vi "Go.vi"(9 "Timing Data":T1(array[cluster]), 10 "Control In":T2={"I-O.lvclass"=refnum, "Gantry"=refnum, "Dispenser"="COM1"}, 11 "C4 Dispense in":refnum<class "Iterative Dispense.lvclass">) -> (2 "Control Out":T2={"I-O.lvclass"=refnum, "Gantry"=refnum, "Dispenser"="COM1"}, 3 "C4 Dispense Out":refnum<class "Iterative Dispense.lvclass">)   [LabVIEW 2018, in "Iterative Dispense.lvclass"]
uses:
  Iterative Dispense.lvclass
  C:/Users/HEP/Documents/GitHub/New folder/C/Users/HEP/Documents/GitHub/UCSB-Gantry-HEP-2018/Classes/Routine/Dispense/Dispense.lvclass
  Controller/Controllers.ctl
  Controller/I-O/I-O.lvclass
  C:/Program Files (x86)/Aerotech/A3200/LabVIEW/2010/Bin/Aerotech.A3200.dll
  Program Files (x86)/Aerotech/A3200/LabVIEW/2010/Bin/Aerotech.A3200.dll
  Iterative Dispense.lvclass/Iterative Dispense.ctl
  Controller/Motion/A3200/A3200.lvclass
  Controller/Dispenser/Dispenser.lvclass
  Controller/Motion/Motion.lvclass
  Controller/Controller.lvclass
panel:
  out "error out":errorcluster
  in  "error in (no error)":errorcluster
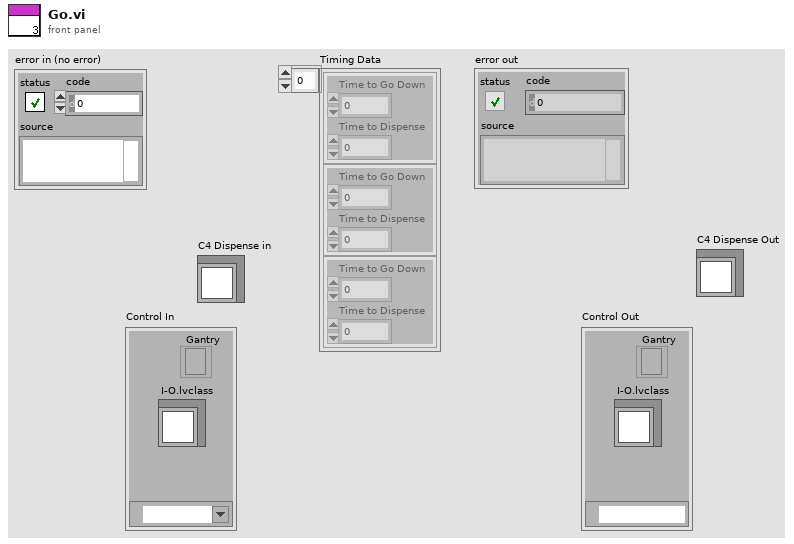
[diagram p1: front panel]
types:
  T1 = cluster{"Time to Go Down":i32, "Time to Dispense":i32}[]
  T2 = typedef "Controller.lvclass/Controllers.ctl" = cluster{"I-O.lvclass":refnum<class "I-O.lvclass">, "Gantry":refnum<k24>, "Dispenser":refnum<visa-resource-name>}
  T3 = typedef "Iterative Dispense.lvclass/Glue Step Enum.ctl" = enum16{"Baseplate to Kapton", "Kapton to Sensor"}
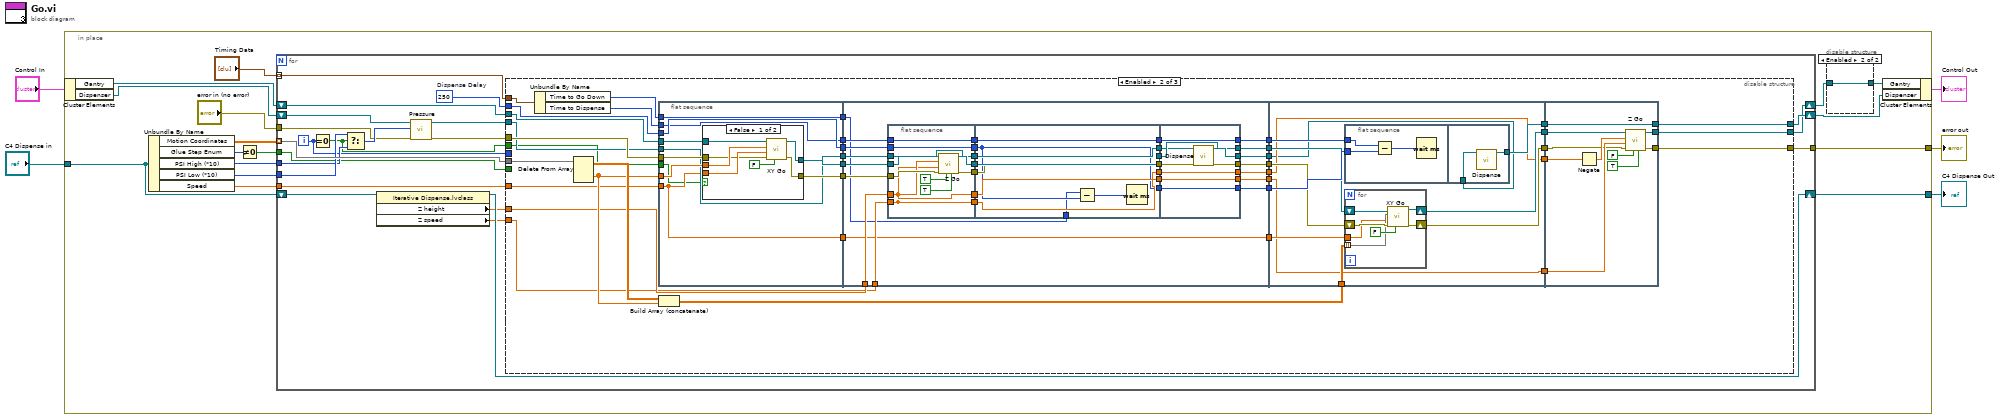
[diagram p0: block diagram]
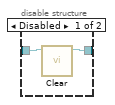
[diagram p2: hidden frame]
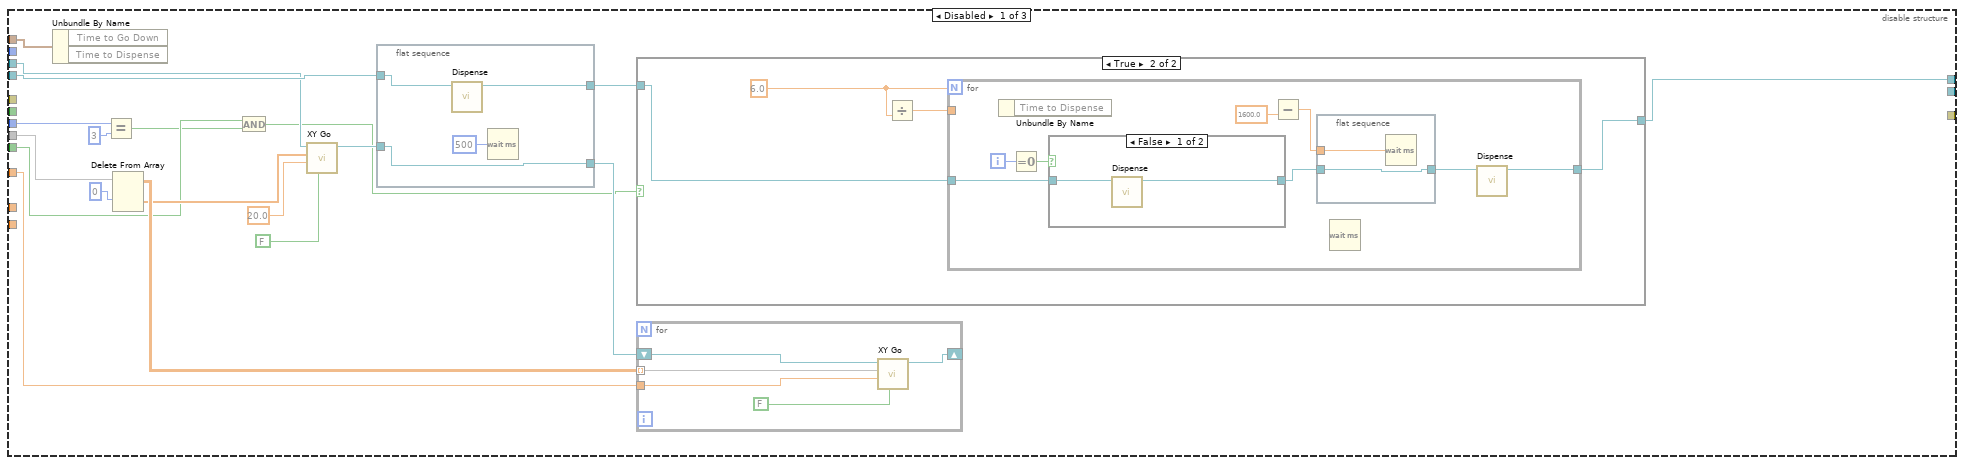
[diagram p3: hidden frame]
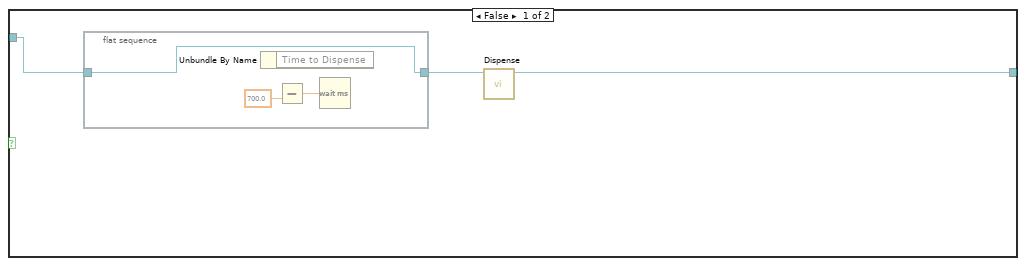
[diagram p4: hidden frame]
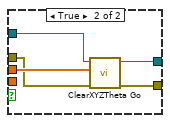
[diagram p6: hidden frame]
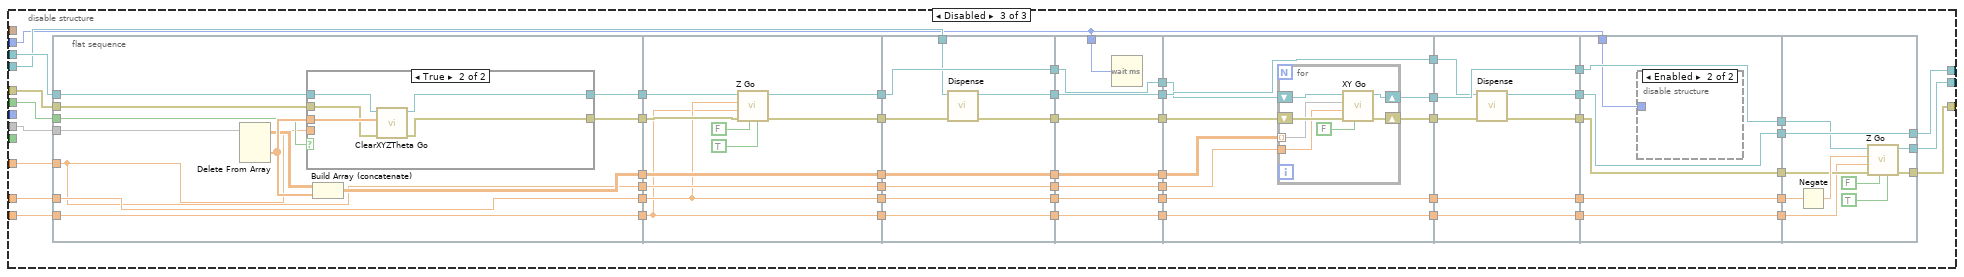
[diagram p7: hidden frame]
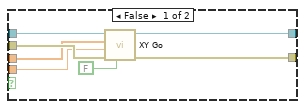
[diagram p8: hidden frame]
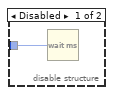
[diagram p9: hidden frame]
diagram:
  n1 = in-place {
    in-place-border: "C4 Dispense in" -> [w9]
    in-place-border: [w10] -> w2
    in-place-border: [w7] -> w1
    n2 = in-place-cluster #1("Control In") -> ("Gantry"=w15:refnum<k24>, "Dispenser"=w13:refnum<visa-resource-name>)
    n3 = Unbundle By Name(w9) -> ("Motion Coordinates"=w17:dbl[][][], "Glue Step Enum"=w16:T3, "PSI High (*10)"=w20:i32, "PSI Low (*10)"=w19:i32, "Speed"=w18:dbl)
    n4 = Not Equal To 0?(x=w16) -> (x != 0?=w21:bool)
    n5 = for {
      tunnel: w17 -> [w45] mode=indexing
      tunnel: w21 -> [w26]
      tunnel: w18 -> [w44]
      tunnel: w19 -> [w43]
      tunnel: w20 -> [w42]
      shift-right: [w28] -> w12
      shift-left: w15 -> [w40]
      shift-right: [w46] -> w14
      shift-left: w13 -> [w39]
      tunnel: "error in (no error)" -> [w36]
      shift-right: [w34] -> w10
      shift-left: w9 -> [w35]
      tunnel: [w30] -> w7
      tunnel: "Timing Data" -> [w27] mode=indexing
      i -> [w25]
      w31 = 250  # Dispense Delay
      # "Executes C4 Symmetric Motion"
      n6 = Equal To 0?(x=w25) -> (x = 0?=w29:bool)
      n7 = Select(t=w43, s=w29, f=w42) -> (s? t:f=w41:i32)
      n8 = property class="Iterative Dispense.lvclass"(reference=w35) -> (reference out=w34:refnum<class "Iterative Dispense.lvclass">, "Z height"=w33:dbl, "Z speed"=w32:dbl)  [unwired: 1 in, 1 out]
      n9 = call "Pressure.vi"("error in (no error)"=w36, "Pressure"=w41, "VISA resource name"=w39) -> ("error out"=w37:errorcluster, "VISA resource name out"=w38:refnum<visa-resource-name>)  [unwired: 7 in]
      n10 = disable-structure shown="Enabled" {
        disable-tunnel: [w65 w109 w285] -> w46
        disable-tunnel: w45 -> [w64 w121 w287]
        disable-tunnel: w44 -> [w59 w118 w304]
        disable-tunnel: w38 -> [w58 w116 w286]
        disable-tunnel: w40 -> [w57 w123 w289]
        disable-tunnel: w37 -> [_ w117 w288]
        disable-tunnel: w33 -> [_ w114 w291]
        disable-tunnel: w32 -> [_ w113 w292]
        disable-tunnel: w31 -> [_ w105 w255]
        disable-tunnel: [_ w108 w284] -> w30
        disable-tunnel: w29 -> [_ w98 w290]
        disable-tunnel: [_ w122 w252] -> w28
        disable-tunnel: w27 -> [w52 w107 _]
        disable-tunnel: w26 -> [w51 _ _]
        disable-tunnel: w25 -> [w50 _ _]
        frame Disabled {
          n11 = Unbundle By Name(w52) -> ()  [unwired: 2 out]
          n12 = Equal?(x=w50, y=3) -> (x = y?=w48:bool)
          n13 = Delete From Array(array=w64, index (row)=0) -> (deleted portion=w55:dbl[], array with subset deleted=w62:dbl[][])  [unwired: 2 in]
          n14 = And(x=w51, y=w48) -> (x .and. y?=w47:bool)
          n15 = call "XY Go.vi"("return immediately"=FALSE, "Speed"=20.0 ("speed"), "XY In"=w55, "Gantry In"=w57) -> ("Gantry Out"=w56:refnum<k24>)  [unwired: 5 in, 2 out]
          n16 = flat-sequence {
            tunnel: w58 -> [w89]
            tunnel: w56 -> [w91]
            tunnel: [w91] -> w61
            tunnel: [w90] -> w60
            frame #0 {
              n17 = call "Dispense.vi"("Dispenser In"=w89) -> ("Dispenser Out"=w90:refnum<visa-resource-name>)  [unwired: 9 in, 1 out]
              n18 = Wait (ms)(milliseconds to wait=u32 500) -> ()  [unwired: 1 out]
            }
          }
          n19 = case shown="True" w47 {
            tunnel: w60 -> [w68 w74]
            tunnel: [w67 w73] -> w65
            frame False {
              n20 = flat-sequence {
                tunnel: w68 -> [w69]
                tunnel: [w69] -> w66
                frame #0 {
                  n21 = Unbundle By Name() -> ()  [unwired: 1 in, 1 out]
                  n22 = Subtract(y=700.0) -> (x-y=w71:dbl)  [unwired: 1 in]
                  n23 = Wait (ms)(milliseconds to wait=w71) -> ()  [unwired: 1 out]
                }
              }
              n24 = call "Dispense.vi"("Dispenser In"=w66) -> ("Dispenser Out"=w67:refnum<visa-resource-name>)  [unwired: 9 in, 1 out]
            }
            frame True {
              w72 = 6.0 ("y")
              # "Leaves Space for Silver Epoxy"
              n25 = Divide(y=w72) -> (x/y=w75:dbl)  [unwired: 1 in]
              n26 = for {
                N: w72 -> [_]
                tunnel: w75 -> [_]
                tunnel: w74 -> [w81]
                tunnel: [w77] -> w73
                i -> [w79]
                n27 = Unbundle By Name() -> ()  [unwired: 1 in, 1 out]
                n28 = Equal To 0?(x=w79) -> (x = 0?=w78:bool)
                n29 = case shown="False" w78 {
                  tunnel: w81 -> [w84 w86]
                  tunnel: [w85 w86] -> w80
                  frame False {
                    n30 = call "Dispense.vi"("Dispenser In"=w84) -> ("Dispenser Out"=w85:refnum<visa-resource-name>)  [unwired: 9 in, 1 out]
                  }
                  frame True {
                  }
                }
                n31 = Subtract(y=1600.0) -> (x-y=w82:dbl)  [unwired: 1 in]
                n32 = flat-sequence {
                  tunnel: w82 -> [w88]
                  tunnel: w80 -> [w87]
                  tunnel: [w87] -> w76
                  frame #0 {
                    n33 = Wait (ms)(milliseconds to wait=w88) -> ()  [unwired: 1 out]
                  }
                }
                n34 = Wait (ms)() -> ()  [unwired: 1 in, 1 out]
                n35 = call "Dispense.vi"("Dispenser In"=w76) -> ("Dispenser Out"=w77:refnum<visa-resource-name>)  [unwired: 9 in, 1 out]
              }
            }
          }
          n36 = for {
            tunnel: w59 -> [w94]
            tunnel: w62 -> [w95] mode=indexing
            shift-right: [w96] -> _
            shift-left: w61 -> [w97]
            n37 = call "XY Go.vi"("return immediately"=FALSE, "Speed"=w94, "XY In"=w95, "Gantry In"=w97) -> ("Gantry Out"=w96:refnum<k24>)  [unwired: 5 in, 2 out]
          }
        }
        frame Enabled {
          n38 = Unbundle By Name(w107) -> ("Time to Go Down"=w102:i32, "Time to Dispense"=w100:i32)
          n39 = Delete From Array(array=w121) -> (deleted portion=w119:dbl[], array with subset deleted=w120:dbl[][])  [unwired: 3 in]
          n40 = flat-sequence {
            tunnel: w123 -> [w146]
            tunnel: [w145] -> w135
            tunnel: [w142] -> w134
            tunnel: w119 -> [w144]
            tunnel: w118 -> [w140]
            tunnel: w117 -> [w143]
            tunnel: w116 -> [w141]
            tunnel: [w141] -> w115
            tunnel: [w140] -> w111
            tunnel: [w139] -> w106
            tunnel: w105 -> [w139]
            tunnel: [w138] -> w103
            tunnel: w102 -> [w138]
            tunnel: [w137] -> w101
            tunnel: w100 -> [w137]
            tunnel: w98 -> [w136]
            tunnel: w135 -> [w187]
            tunnel: [w188] -> w133
            tunnel: [w186] -> w132
            tunnel: w134 -> [w185]
            tunnel: [w183] -> w131
            tunnel: [w182] -> w130
            tunnel: [w181] -> w129
            tunnel: w115 -> [w184]
            tunnel: w114 -> [w180]
            tunnel: w113 -> [w179]
            tunnel: w111 -> [w178]
            tunnel: [w178] -> w110
            tunnel: w106 -> [w177]
            tunnel: [w176] -> w104
            tunnel: w103 -> [w159]
            tunnel: w101 -> [w175]
            tunnel: [w174] -> w99
            tunnel: w133 -> [w218]
            tunnel: [w229] -> w128
            tunnel: w132 -> [w226]
            tunnel: [w222] -> w127
            tunnel: [w220] -> w126
            tunnel: w131 -> [w220]
            tunnel: [w219] -> w125
            tunnel: w130 -> [w219]
            tunnel: w129 -> [w225]
            tunnel: [w221] -> w124
            tunnel: w112 -> [w224]
            tunnel: w110 -> [w223]
            tunnel: w104 -> [w228]
            tunnel: w99 -> [w227]
            tunnel: [w251] -> w122
            tunnel: w128 -> [w250]
            tunnel: [w250] -> w109
            tunnel: w127 -> [w249]
            tunnel: [w248] -> w108
            tunnel: w126 -> [w247]
            tunnel: w125 -> [w245]
            tunnel: w124 -> [w242]
            frame #0 {
              n41 = case shown="False" w136 {
                tunnel: w146 -> [w153 w158]
                tunnel: [w152 w157] -> w145
                tunnel: [w151 w156] -> w142
                tunnel: w144 -> [w149 w155]
                tunnel: w140 -> [w148 _]
                tunnel: w143 -> [w147 w154]
                frame False {
                  n42 = call "XY Go.vi"("return immediately"=FALSE, "error in (no error)"=w147, "Speed"=w148, "XY In"=w149, "Gantry In"=w153) -> ("error out"=w151:errorcluster, "Gantry Out"=w152:refnum<k24>)  [unwired: 4 in, 1 out]
                }
                frame True {
                  n43 = call "ClearXYZTheta Go.vi"("error in (no error)"=w154, "XYZTheta In"=w155, "Gantry In"=w158) -> ("error out"=w156:errorcluster, "Gantry Out"=w157:refnum<k24>)  [unwired: 6 in, 1 out]
                }
              }
            }
            frame #1 {
              n44 = flat-sequence {
                tunnel: w187 -> [w199]
                tunnel: [w197] -> w173
                tunnel: w185 -> [w194]
                tunnel: [w196] -> w171
                tunnel: w184 -> [w196]
                tunnel: [w189] -> w169
                tunnel: [w193] -> w167
                tunnel: w180 -> [w190]
                tunnel: w179 -> [w189]
                tunnel: [w192] -> w165
                tunnel: w177 -> [w192]
                tunnel: w175 -> [w191]
                tunnel: [w191] -> w163
                tunnel: [w190] -> w161
                tunnel: w173 -> [w208]
                tunnel: [w208] -> w172
                tunnel: w171 -> [w207]
                tunnel: [w207] -> w170
                tunnel: w169 -> [w206]
                tunnel: [w206] -> w168
                tunnel: w167 -> [w205]
                tunnel: [w205] -> w166
                tunnel: w165 -> [w202]
                tunnel: [w202] -> w164
                tunnel: w163 -> [w204]
                tunnel: [w204] -> w162
                tunnel: w161 -> [w203]
                tunnel: [w203] -> w160
                tunnel: w159 -> [w201]
                tunnel: [w217] -> w188
                tunnel: w172 -> [w216]
                tunnel: [w216] -> w186
                tunnel: w170 -> [w215]
                tunnel: [w214] -> w183
                tunnel: [w213] -> w182
                tunnel: w168 -> [w213]
                tunnel: w166 -> [w212]
                tunnel: [w211] -> w181
                tunnel: [w210] -> w176
                tunnel: w164 -> [w210]
                tunnel: [w209] -> w174
                tunnel: w162 -> [w209]
                tunnel: w160 -> [w214]
                frame #0 {
                  n45 = call "Z Go.vi"("Increment"=TRUE, "Return Immediately"=TRUE, "error in (no error)"=w194, "Speed In"=w189, "Position In"=w190, "Gantry In"=w199) -> ("error out"=w193:errorcluster, "Gantry Out"=w197:refnum<k24>)  [unwired: 2 in, 2 out]
                }
                frame #1 {
                  n46 = Subtract(x=w201, y=w202) -> (x-y=w200:i32)
                  n47 = Wait (ms)(milliseconds to wait=w200) -> ()  [unwired: 1 out]
                }
                frame #2 {
                  n48 = call "Dispense.vi"("error in (no error)"=w212, "Dispenser In"=w215) -> ("error out"=w211:errorcluster, "Dispenser Out"=w217:refnum<visa-resource-name>)  [unwired: 8 in]
                }
              }
            }
            frame #2 {
              n49 = flat-sequence {
                tunnel: w228 -> [w239]
                tunnel: w227 -> [w238]
                tunnel: [w241] -> w229
                tunnel: w218 -> [w240]
                frame #0 {
                  n50 = Subtract(x=w238, y=w239) -> (x-y=w237:i32)
                  n51 = Wait (ms)(milliseconds to wait=w237) -> ()  [unwired: 1 out]
                }
                frame #1 {
                  n52 = call "Dispense.vi"("Dispenser In"=w240) -> ("Dispenser Out"=w241:refnum<visa-resource-name>)  [unwired: 9 in, 1 out]
                }
              }
              n53 = for {
                shift-right: [w234] -> w222
                shift-left: w226 -> [w235]
                shift-right: [w232] -> w221
                shift-left: w225 -> [w233]
                tunnel: w224 -> [w231] mode=indexing
                tunnel: w223 -> [w230]
                n54 = call "XY Go.vi"("return immediately"=FALSE, "error in (no error)"=w233, "Speed"=w230, "XY In"=w231, "Gantry In"=w235) -> ("error out"=w232:errorcluster, "Gantry Out"=w234:refnum<k24>)  [unwired: 4 in, 1 out]
              }
            }
            frame #3 {
              n55 = Negate(x=w247) -> (-x=w246:dbl)
              n56 = call "Z Go.vi"("Increment"=TRUE, "Return Immediately"=FALSE, "error in (no error)"=w242, "Speed In"=w245, "Position In"=w246, "Gantry In"=w249) -> ("error out"=w248:errorcluster, "Gantry Out"=w251:refnum<k24>)  [unwired: 2 in, 2 out]
            }
          }
          n57 = Build Array (concatenate)(w120, w119) -> (w112:dbl[][])
        }
        frame Disabled {
          n58 = flat-sequence {
            tunnel: w292 -> [w315]
            tunnel: w291 -> [w316]
            tunnel: [w308] -> w303
            tunnel: [w307] -> w302
            tunnel: [w316] -> w301
            tunnel: [w315] -> w300
            tunnel: w290 -> [w312]
            tunnel: w289 -> [w311]
            tunnel: w288 -> [w310]
            tunnel: w304 -> [w305]
            tunnel: w287 -> [w309]
            tunnel: [w306] -> w283
            tunnel: [w305] -> w281
            tunnel: [w336] -> w299
            tunnel: [w333] -> w298
            tunnel: w303 -> [w338]
            tunnel: w302 -> [w334]
            tunnel: w301 -> [w330]
            tunnel: w300 -> [w329]
            tunnel: w283 -> [w332]
            tunnel: [w332] -> w282
            tunnel: w281 -> [w331]
            tunnel: [w331] -> w280
            tunnel: [w330] -> w254
            tunnel: [w329] -> w253
            tunnel: w299 -> [w346]
            tunnel: w298 -> [w343]
            tunnel: w286 -> [w341]
            tunnel: [w347] -> w279
            tunnel: [w346] -> w277
            tunnel: [w345] -> w275
            tunnel: [w344] -> w273
            tunnel: [w342] -> w271
            tunnel: w282 -> [w340]
            tunnel: [w340] -> w269
            tunnel: w280 -> [w339]
            tunnel: [w339] -> w267
            tunnel: w254 -> [w345]
            tunnel: w253 -> [w344]
            tunnel: w279 -> [w355]
            tunnel: [w355] -> w278
            tunnel: w277 -> [w354]
            tunnel: [w354] -> w276
            tunnel: w275 -> [w353]
            tunnel: [w353] -> w274
            tunnel: w273 -> [w352]
            tunnel: [w352] -> w272
            tunnel: w271 -> [w351]
            tunnel: [w351] -> w270
            tunnel: w269 -> [w350]
            tunnel: [w350] -> w268
            tunnel: w267 -> [w349]
            tunnel: [w349] -> w266
            tunnel: w255 -> [w348]
            tunnel: w278 -> [w364]
            tunnel: w276 -> [w361]
            tunnel: w274 -> [w363]
            tunnel: w272 -> [w362]
            tunnel: w270 -> [w359]
            tunnel: [w364] -> w297
            tunnel: [w360] -> w296
            tunnel: [w363] -> w295
            tunnel: [w362] -> w294
            tunnel: [w358] -> w293
            tunnel: w268 -> [w357]
            tunnel: w266 -> [w356]
            tunnel: w297 -> [w373]
            tunnel: w296 -> [w378]
            tunnel: w295 -> [w377]
            tunnel: w294 -> [w376]
            tunnel: w293 -> [w375]
            tunnel: [w372] -> w265
            tunnel: [w378] -> w263
            tunnel: [w377] -> w261
            tunnel: [w376] -> w259
            tunnel: [w374] -> w257
            tunnel: w265 -> [w384]
            tunnel: [w384] -> w264
            tunnel: w263 -> [w383]
            tunnel: [w383] -> w262
            tunnel: w261 -> [w382]
            tunnel: [w382] -> w260
            tunnel: w259 -> [w381]
            tunnel: [w381] -> w258
            tunnel: w257 -> [w380]
            tunnel: [w380] -> w256
            tunnel: w255 -> [w379]
            tunnel: [w390] -> w252
            tunnel: [w395] -> w285
            tunnel: w264 -> [w395]
            tunnel: w262 -> [w391]
            tunnel: w260 -> [w387]
            tunnel: w258 -> [w386]
            tunnel: w256 -> [w389]
            tunnel: [w388] -> w284
            frame #0 {
              n59 = Delete From Array(array=w309) -> (deleted portion=w314:dbl[], array with subset deleted=w313:dbl[][])  [unwired: 3 in]
              n60 = case shown="True" w312 {
                tunnel: [w322 w328] -> w308
                tunnel: [w321 w327] -> w307
                tunnel: w314 -> [w317 w326]
                tunnel: w311 -> [w323 w325]
                tunnel: w310 -> [w319 w324]
                tunnel: w305 -> [w318 _]
                frame False {
                  n61 = call "XY Go.vi"("return immediately"=FALSE, "error in (no error)"=w319, "Speed"=w318, "XY In"=w317, "Gantry In"=w323) -> ("error out"=w321:errorcluster, "Gantry Out"=w322:refnum<k24>)  [unwired: 4 in, 1 out]
                }
                frame True {
                  n62 = call "ClearXYZTheta Go.vi"("error in (no error)"=w324, "XYZTheta In"=w326, "Gantry In"=w325) -> ("error out"=w327:errorcluster, "Gantry Out"=w328:refnum<k24>)  [unwired: 6 in, 1 out]
                }
              }
              n63 = Build Array (concatenate)(w313, w314) -> (w306:dbl[][])
            }
            frame #1 {
              n64 = call "Z Go.vi"("Increment"=TRUE, "Return Immediately"=FALSE, "error in (no error)"=w334, "Speed In"=w329, "Position In"=w330, "Gantry In"=w338) -> ("error out"=w333:errorcluster, "Gantry Out"=w336:refnum<k24>)  [unwired: 2 in, 2 out]
            }
            frame #2 {
              n65 = call "Dispense.vi"("error in (no error)"=w343, "Dispenser In"=w341) -> ("error out"=w342:errorcluster, "Dispenser Out"=w347:refnum<visa-resource-name>)  [unwired: 8 in]
            }
            frame #3 {
              n66 = Wait (ms)(milliseconds to wait=w348) -> ()  [unwired: 1 out]
            }
            frame #4 {
              n67 = for {
                shift-right: [w369] -> w360
                shift-left: w361 -> [w370]
                shift-right: [w367] -> w358
                shift-left: w359 -> [w368]
                tunnel: w357 -> [w366] mode=indexing
                tunnel: w356 -> [w365]
                n68 = call "XY Go.vi"("return immediately"=FALSE, "error in (no error)"=w368, "Speed"=w365, "XY In"=w366, "Gantry In"=w370) -> ("error out"=w367:errorcluster, "Gantry Out"=w369:refnum<k24>)  [unwired: 4 in, 1 out]
              }
            }
            frame #5 {
              n69 = call "Dispense.vi"("error in (no error)"=w375, "Dispenser In"=w373) -> ("error out"=w374:errorcluster, "Dispenser Out"=w372:refnum<visa-resource-name>)  [unwired: 8 in]
            }
            frame #6 {
              n70 = disable-structure shown="Enabled" {
                disable-tunnel: w379 -> [w385 _]
                frame Disabled {
                  n71 = Wait (ms)(milliseconds to wait=w385) -> ()  [unwired: 1 out]
                }
                frame Enabled {
                }
              }
            }
            frame #7 {
              n72 = Negate(x=w387) -> (-x=w394:dbl)
              n73 = call "Z Go.vi"("Increment"=TRUE, "Return Immediately"=FALSE, "error in (no error)"=w389, "Speed In"=w386, "Position In"=w394, "Gantry In"=w391) -> ("error out"=w388:errorcluster, "Gantry Out"=w390:refnum<k24>)  [unwired: 2 in, 2 out]
            }
          }
        }
      }
    }
    n74 = disable-structure shown="Enabled" {
      disable-tunnel: w12 -> [w23 w24]
      disable-tunnel: [w22 w24] -> w11
      frame Disabled {
        n75 = call "Clear.vi"("Gantry In"=w23) -> ("Gantry Out"=w22:refnum<k24>)  [unwired: 9 in, 1 out]
      }
      frame Enabled {
      }
    }
    n76 = in-place-cluster #1("Gantry"=w11, "Dispenser"=w14) -> (→"Control Out":T2)
  }
  "C4 Dispense Out" <- w2
  "error out" <- w1
